vi "ZoomOnPeak.vi"(6 "Now.Target":T1=enum."4", 8 "Quadrature spectrum in":dbl[](array[numeric]), 9 "InPhase spectrum in":dbl[](array[numeric]), 10 "ZoomWidth":i32=20, 11 "Power spectrum in":dbl[](array[numeric])) -> (0 "ZoomSpectrs":T2, 1 "Power of Peak":dbl, 2 "MaxIndex":i32, 3 "ZoomQ":cluster{"ZoomQPos":dbl[], "ZoomQNeg":dbl[]}, 5 "ZoomI":cluster{"ZoomIPos":dbl[], "ZoomINeg":dbl[]}, 7 "PeakValues":cluster{"IN":dbl, "IP":dbl, "QN":dbl, "QP":dbl})   [LabVIEW 2018]
uses:
  Controls/Clusts/ZoomSpectrumsClust.ctl
  Controls/Enums/TargetNumber.ctl
  <vilib>/ptbypt/NI_PtbyPt.lvlib
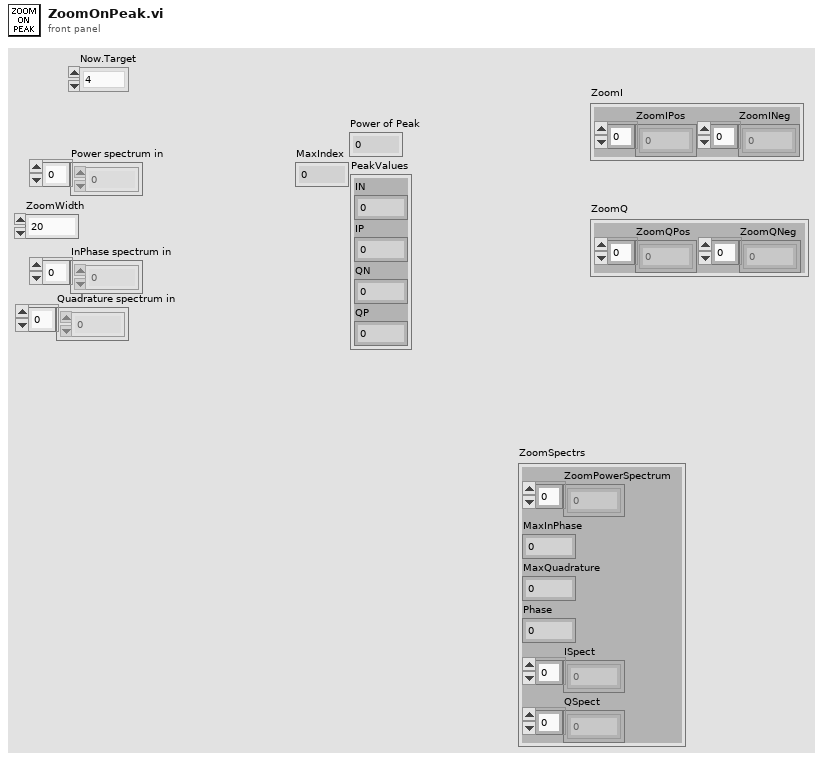
[diagram p1: front panel]
types:
  T1 = typedef "TargetNumber.ctl" = enum16{"1", "2", "3", "4"}
  T2 = typedef "ZoomSpectrumsClust.ctl" = cluster{"ZoomPowerSpectrum":dbl[], "MaxInPhase":dbl, "MaxQuadrature":dbl, "Phase":dbl, "ISpect":dbl[], "QSpect":dbl[]}
  T3 = cluster{"ZoomSpectrumPos":dbl[], "ZoomSpectrumNeg":dbl[]}
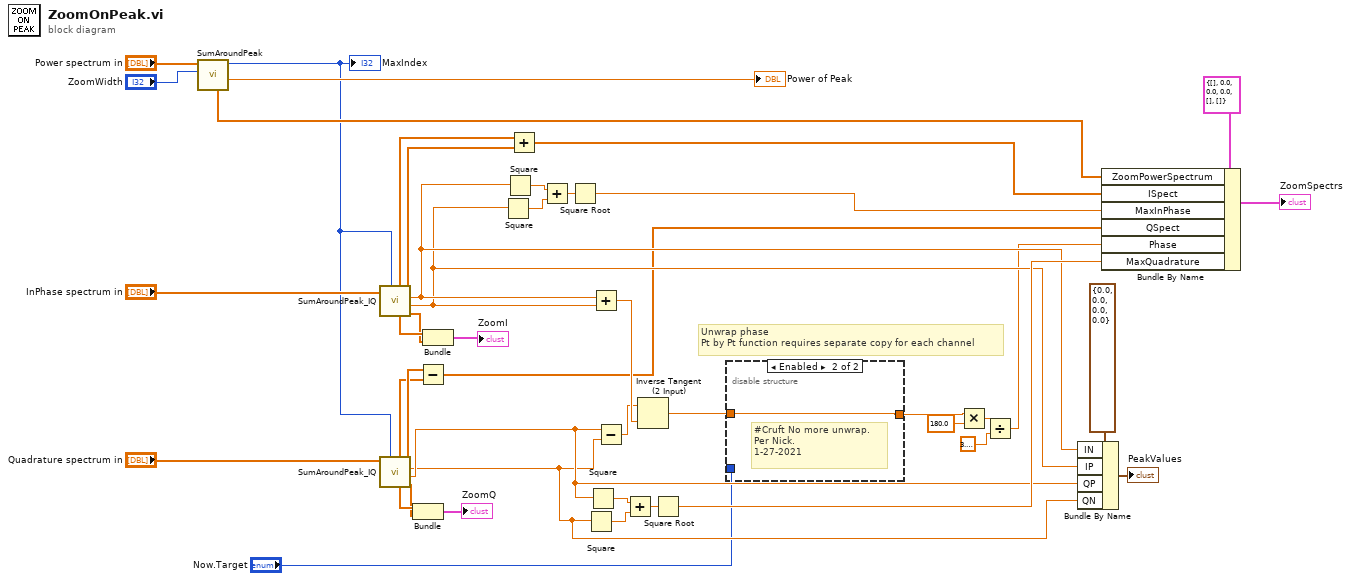
[diagram p0: block diagram]
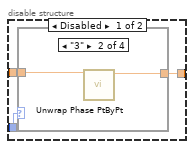
[diagram p2: hidden frame]
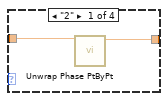
[diagram p3: hidden frame]
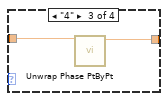
[diagram p4: hidden frame]
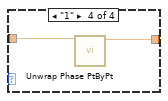
[diagram p5: hidden frame]
diagram:
  # "Unwrap phase\nPt by Pt function requires separate copy for each channel"
  n1 = call "SumAroundPeak.vi"("ZoomWidth"="ZoomWidth", "spectrum in"="Power spectrum in") -> ("SumOfPeak"=→"Power of Peak":dbl, "MaxIndex"=w36:i32, "ZoomSpectrum"=w38:dbl[])  [unwired: 6 in, 1 out]
  "MaxIndex" <- w36
  n2 = call "SumAroundPeak_IQ.vi"("MaxIndex"=w36, "spectrum in"="InPhase spectrum in") -> ("ZoomSpectrumNeg"=w15:dbl[], "Positive Max"=w20:dbl, "Negative_Max"=w21:dbl, "PosZoomSpect"=w5:dbl[], "ZoomSpectrumPos"=w16:dbl[], "NegZoomSpect"=w6:dbl[])  [unwired: 4 in]
  n3 = call "SumAroundPeak_IQ.vi"("MaxIndex"=w36, "spectrum in"="Quadrature spectrum in") -> ("ZoomSpectrumNeg"=w12:dbl[], "Positive Max"=w19:dbl, "Negative_Max"=w18:dbl, "PosZoomSpect"=w3:dbl[], "ZoomSpectrumPos"=w13:dbl[], "NegZoomSpect"=w2:dbl[])  [unwired: 4 in]
  n4 = Bundle("ZoomSpectrumPos"=w13, "ZoomSpectrumNeg"=w12) -> (→"ZoomQ":T3)  [unwired: 1 in]
  n5 = Subtract(x=w3, y=w2) -> (x-y=w1:dbl[])
  n6 = Bundle("ZoomSpectrumPos"=w16, "ZoomSpectrumNeg"=w15) -> (→"ZoomI":T3)  [unwired: 1 in]
  n7 = Square(x=w20) -> (x^2=w29:dbl)
  n8 = Square(x=w21) -> (x^2=w30:dbl)
  n9 = Add(x=w6, y=w5) -> (x+y=w4:dbl[])
  n10 = Add(x=w30, y=w29) -> (x+y=w28:dbl)
  n11 = Square Root(x=w28) -> (sqrt(x)=w27:dbl)
  n12 = Square(x=w18) -> (x^2=w25:dbl)
  n13 = Square(x=w19) -> (x^2=w24:dbl)
  n14 = Add(x=w21, y=w20) -> (x+y=w32:dbl)
  n15 = Subtract(x=w19, y=w18) -> (x-y=w31:dbl)
  n16 = Add(x=w24, y=w25) -> (x+y=w26:dbl)
  n17 = Inverse Tangent (2 Input)(1:w32, 2:w31) -> (0:w9:dbl)
  n18 = Square Root(x=w26) -> (sqrt(x)=w23:dbl)
  n19 = disable-structure shown="Enabled" {
    disable-tunnel: w9 -> [w47 w56]
    disable-tunnel: [w46 w56] -> w8
    disable-tunnel: "Now.Target" -> [w45 _]
    frame Disabled {
      n20 = case shown="\"3\"" w45 {
        tunnel: w47 -> [w49 w51 w53 w55]
        tunnel: [w48 w50 w52 w54] -> w46
        frame "2" {
          n21 = call <vilib>:"Unwrap Phase PtByPt.vi"("phase"=w49) -> ("unwrapped phase"=w48:dbl)  [unwired: 10 in]
        }
        frame "3" {
          n22 = call <vilib>:"Unwrap Phase PtByPt.vi"("phase"=w51) -> ("unwrapped phase"=w50:dbl)  [unwired: 10 in]
        }
        frame "4" {
          n23 = call <vilib>:"Unwrap Phase PtByPt.vi"("phase"=w53) -> ("unwrapped phase"=w52:dbl)  [unwired: 10 in]
        }
        frame "1" {
          n24 = call <vilib>:"Unwrap Phase PtByPt.vi"("phase"=w55) -> ("unwrapped phase"=w54:dbl)  [unwired: 10 in]
        }
      }
    }
    frame Enabled {
      # "#Cruft No more unwrap.\nPer Nick.\n1-27-2021"
    }
  }
  n25 = Multiply(x=w8, y=180.0) -> (x*y=w35:dbl)
  n26 = Divide(x=w35, y=3.141592653589793) -> (x/y=w10:dbl)
  n27 = Bundle By Name(cluster=cluster{"IN":dbl, "IP":dbl, "QN":dbl, "QP":dbl} {"IN"=0.0, "IP"=0.0, "QN"=0.0, "QP"=0.0}, "IN"=w21, "IP"=w20, "QP"=w19, "QN"=w18) -> (→"PeakValues":cluster{"IN":dbl, "IP":dbl, "QN":dbl, "QP":dbl})
  n28 = Bundle By Name(cluster=T2 {"ZoomPowerSpectrum"=[], "MaxInPhase"=0.0, "MaxQuadrature"=0.0, "Phase"=0.0, "ISpect"=[], "QSpect"=[]} ("ZoomSpectrs"), "ZoomPowerSpectrum"=w38, "ISpect"=w4, "MaxInPhase"=w27, "QSpect"=w1, "Phase"=w10, "MaxQuadrature"=w23) -> (→"ZoomSpectrs":T2)
